vi "GetLogFiles.vi"(7 "LabVIEW Web Service Request":refnum<class "Web Request.lvclass">) -> ()   [LabVIEW 2015]
uses:
  <vilib>/wsapi/Web Request.lvclass
  <vilib>/addons/InsightCM/Utilities/GlobalConfiguration/GlobalConfiguration.lvlib
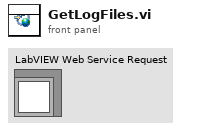
[diagram p1: front panel]
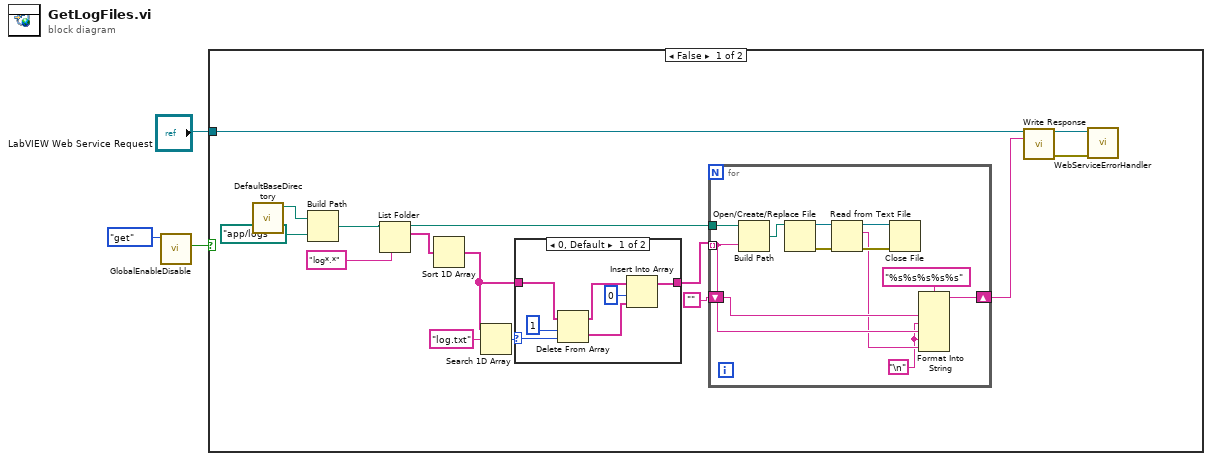
[diagram p0: block diagram]
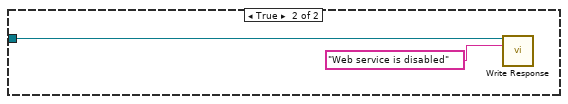
[diagram p3: hidden frame]
diagram:
  n1 = call "GlobalEnableDisable.vi"("action"=enum16{"init", "set", "get"}."get") -> ("DisableDeviceWebService"=w3:bool)  [unwired: 10 in]
  n2 = case shown="False" w3 {
    tunnel: "LabVIEW Web Service Request" -> [w4 w40]
    frame False {
      n3 = call <vilib>:"DefaultBaseDirectory.vi"() -> ("base directory"=w11:path)  [unwired: 11 in]
      n4 = Build Path(base path=w11, name or relative path=path "app/logs" ("base directory")) -> (appended path=w10:path)
      n5 = List Folder(path=w10, pattern="log*.*" ("name or relative path")) -> (path out=w14:path, filenames=w15:string[])  [unwired: 2 in, 2 out]
      n6 = Sort 1D Array(array=w15) -> (sorted array=w6:string[])
      n7 = Search 1D Array(1D array=w6, element="log.txt") -> (index of element=w7:i32)  [unwired: 1 in]
      n8 = case shown="0, Default" w7 {
        selector: w7 -> [w24 _]
        tunnel: w6 -> [w25 w26]
        tunnel: [w19 w26] -> w5
        frame 0, Default {
          n9 = Delete From Array(array=w25, length=1 ("index"), index=w24) -> (deleted portion=w21:string[], array with subset deleted=w22:string[])
          n10 = Insert Into Array(array=w22, index=0, new element=w21) -> (w19:string[])
        }
        frame -1 {
        }
      }
      n11 = for {
        tunnel: w5 -> [w29] mode=indexing
        tunnel: w14 -> [w33]
        shift-right: [w30] -> w12
        shift-left: "" -> [w31]
        w27 = "\n"
        n12 = Build Path(base path=w33, name or relative path=w29) -> (appended path=w34:path)
        n13 = Open/Create/Replace File(file path (use dialog)=w34) -> (refnum out=w38:refnum<file>, error out=w36:errorcluster)  [unwired: 5 in, 1 out]
        n14 = Read from Text File(file (use dialog)=w38, error in=w36) -> (refnum out=w37:refnum<file>, text=w28:string, error out=w35:errorcluster)  [unwired: 2 in, 1 out]
        n15 = Close File(refnum=w37, error in=w35) -> ()  [unwired: 2 out]
        n16 = Format Into String(format string="%s%s%s%s%s", w31, w27, w29, w27, w28) -> (resulting string=w30:string)  [unwired: 2 in, 1 out]
      }
      n17 = call <vilib>:"Write Response.vi"("LabVIEW Web Service Request"=w4, "response string"=w12) -> ("LabVIEW Web Service Request out"=w18:refnum<class "Web Request.lvclass">, "error out"=w17:errorcluster)  [unwired: 12 in]
      n18 = call "WebServiceErrorHandler.vi"("LabVIEW Web Service Request"=w18, "error in (no error)"=w17) -> ()  [unwired: 12 in, 2 out]
    }
    frame True {
      n19 = call <vilib>:"Write Response.vi"("LabVIEW Web Service Request"=w40, "response string"="Web service is disabled") -> ()  [unwired: 12 in, 2 out]
    }
  }
